vi "Update Enable State.vi"(8 "error in (no error)":errorcluster, 11 "Execution UI In":refnum<class "Execution UI.lvclass">) -> (0 "error out":errorcluster, 3 "Execution UI Out":refnum<class "Execution UI.lvclass">)   [LabVIEW 2020, in "Execution UI.lvclass"]
uses:
  Execution UI.lvclass
  C:/git/astemes-lunit/source/User Interface/Process/Process.lvclass
  Process/Process.lvclass/Process.ctl
  Process/Process.lvclass
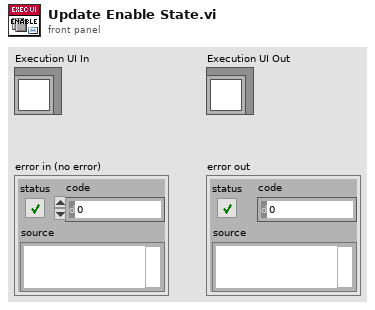
[diagram p1: front panel]
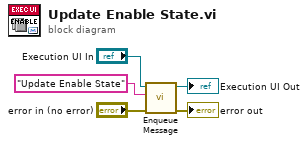
[diagram p0: block diagram]
diagram:
  n1 = call "Enqueue Message.vi"("error in (no error)"="error in (no error)", "Message"="Update Enable State", "Process In"="Execution UI In") -> ("error out"=→"error out":errorcluster, "Process Out"=→"Execution UI Out":refnum<class "Execution UI.lvclass">)  [unwired: 7 in]
